vi "ZyklussteuerungGV.vi"(1 "Zeitpunkte/SPs":T2 {"FPGAPID"."proportional gain (Kc)" format="%.11g"; "FPGAPID"."integral gain (Kc*Ts/Ti)" format="%.11g"; "FPGAPID"."derivative gain (Kc*Td/Ts)" format="%.11g"; "FPGAFixp" format="%.14g"}, 2 "DIOsNummern":cluster{"DIOsMod2BNr":i32[]}[](array[cluster]), 3 "Schieberegister":T1, 6 "FPGA VI Reference In":refnum<k20>) -> (0 "Schieberegister":T1)   [LabVIEW 2010]
uses:
  <vilib>/rvi/errors/niLvFpgaWhatHappensToTopLevelVI.ctl
  <vilib>/rvi/interface/common/niFpgaNodeNameForErrorReporting.ctl
  <vilib>/rvi/errors/niLvFpgaAdjustHostInterfaceError.vi
  <vilib>/rvi/interface/nirviReadWriteControl/nirviReadWriteControl.xnode
  C:/Users/HAGAR-IV/Desktop/Zeugs/markus/version feb 2012/FPGA Bitfiles/pertrasgcfpga2_FPGATarget_FPGA-Programm-10_16368CB6.lvbitx
  C:/Users/HAGAR-IV/Desktop/Zeugs/Johnny/pertrasgc fpga/FPGA-Programm-10-14.vi
  GVZwangs.vi
  GVHorstSP.vi
  GVHeizenLH.vi
  GVVentilposition.vi
  GVZeitenZyklen.vi
  NiFpgaLv.dll
  <vilib>/Utility/error.llb/Error Cluster From Error Code.vi
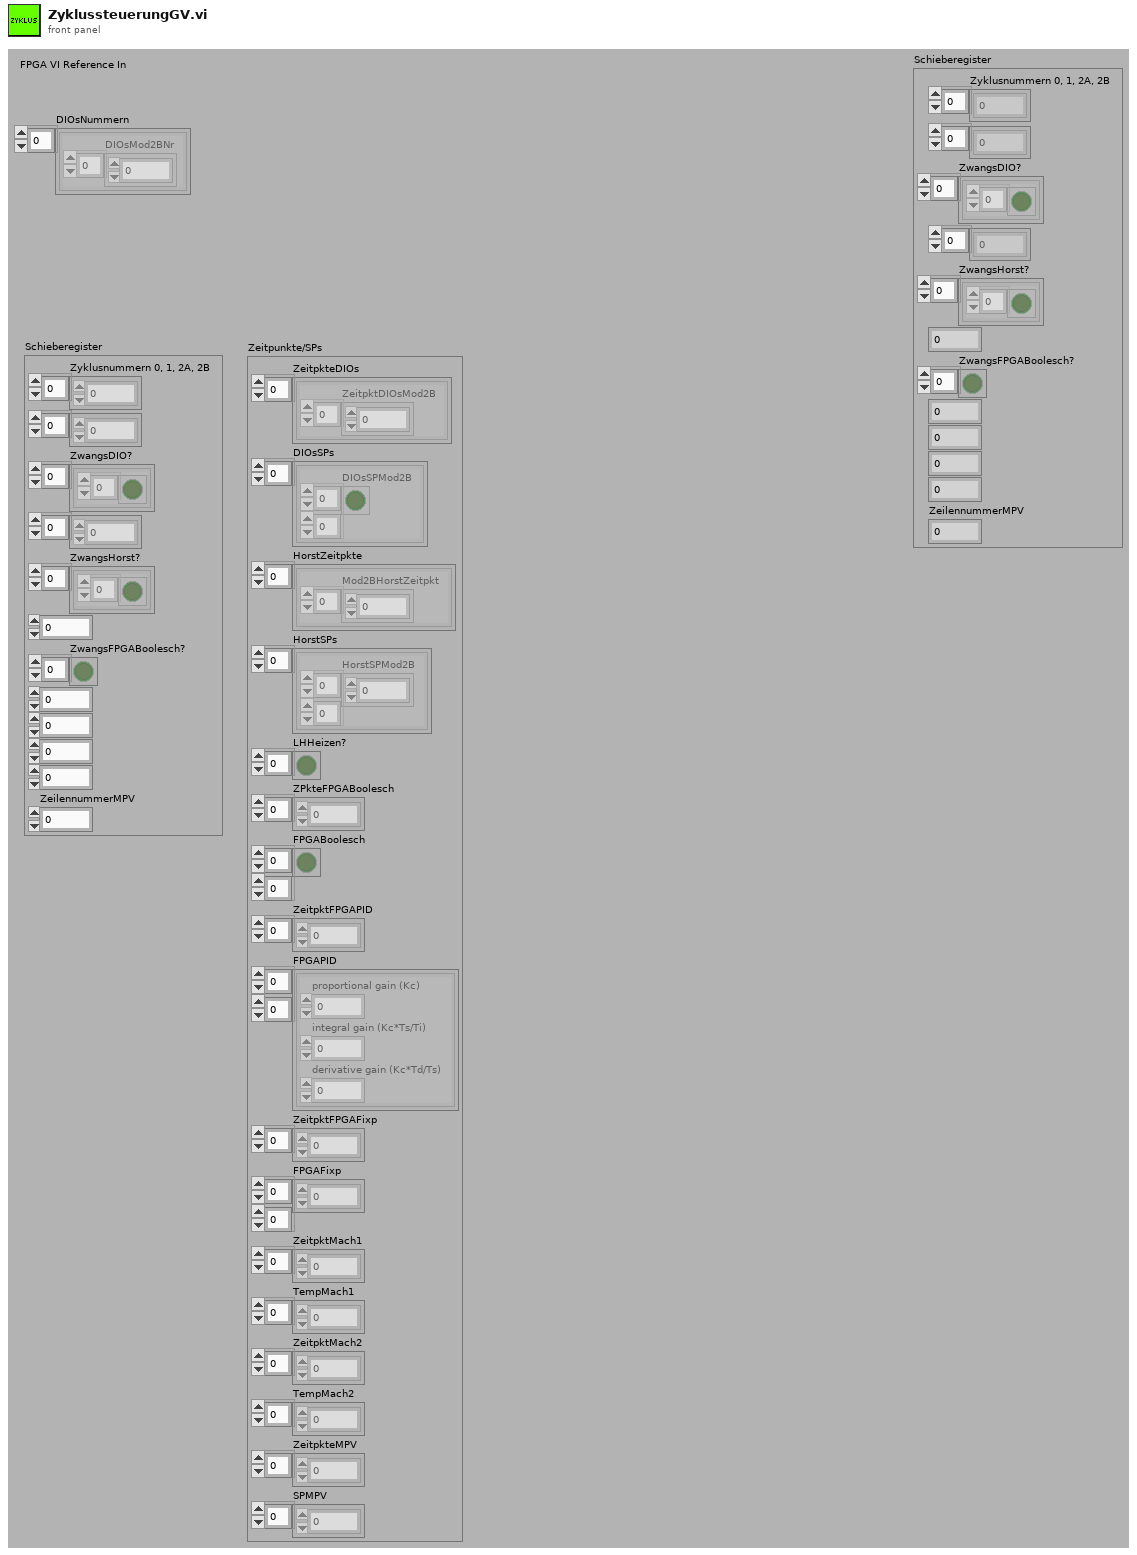
[diagram p1: front panel]
types:
  T1 = cluster{"Zyklusnummern 0, 1, 2A, 2B":i32[], i32[], "ZwangsDIO?":cluster{bool[]}[], i32[], "ZwangsHorst?":cluster{bool[]}[], i32, "ZwangsFPGABoolesch?":bool[], i32, i32, i32, i32, "ZeilennummerMPV":i32}
  T2 = cluster{"ZeitpkteDIOs":cluster{"ZeitpktDIOsMod2B":dbl[]}[], "DIOsSPs":cluster{"DIOsSPMod2B":bool[][]}[], "HorstZeitpkte":cluster{"Mod2BHorstZeitpkt":dbl[]}[], "HorstSPs":cluster{"HorstSPMod2B":dbl[][]}[], "LHHeizen?":bool[], "ZPkteFPGABoolesch":dbl[], "FPGABoolesch":bool[][], "ZeitpktFPGAPID":dbl[], "FPGAPID":cluster{"proportional gain (Kc)":fxp<+/-,16,8>, "integral gain (Kc*Ts/Ti)":fxp<+/-,16,8>, "derivative gain (Kc*Td/Ts)":fxp<+/-,16,8>}[][], "ZeitpktFPGAFixp":dbl[], "FPGAFixp":fxp<+/-,16,4>[][], "ZeitpktMach1":dbl[], "TempMach1":dbl[], "ZeitpktMach2":dbl[], "TempMach2":dbl[], "ZeitpkteMPV":dbl[], "SPMPV":i32[]}
  T3 = cluster{"proportional gain (Kc)":fxp<+/-,16,8>, "integral gain (Kc*Ts/Ti)":fxp<+/-,16,8>, "derivative gain (Kc*Td/Ts)":fxp<+/-,16,8>}[][]
  T4 = typedef "niFpgaNodeNameForErrorReporting.ctl" = enum16{"Open FPGA VI Reference", "Read/Write Control", "Invoke Method: Abort", "Invoke Method: Acknowledge IRQ", "Invoke Method: Download", "Invoke Method: FIFO.Configure", "Invoke Method: FIFO.Read", "Invoke Method: FIFO.Start", "Invoke Method: FIFO.Stop", "Invoke Method: FIFO.Write", "Invoke Method: Reset", "Invoke Method: Run", "Invoke Method: Wait on IRQ", "Close FPGA VI Reference"}
  T5 = typedef "niLvFpgaWhatHappensToTopLevelVI.ctl" = enum16{"top level VI scripted behind XNode", "top level VI inlined behind XNode"}
  T6 = cluster{"FPGAFixp[0]":fxp<+/-,16,4>, "FPGAFixp[1]":fxp<+/-,16,4>, "FPGAFixp[2]":fxp<+/-,16,4>, "FPGAFixp[3]":fxp<+/-,16,4>, "FPGAFixp[4]":fxp<+/-,16,4>, "FPGAFixp[5]":fxp<+/-,16,4>, "FPGAFixp[6]":fxp<+/-,16,4>, "FPGAFixp[7]":fxp<+/-,16,4>}
  T7 = cluster{"proportional gain (Kc)":fxp<+/-,16,8>, "integral gain (Kc*Ts/Ti)":fxp<+/-,16,8>, "derivative gain (Kc*Td/Ts)":fxp<+/-,16,8>}[]
  T8 = cluster{"FPGAPID[0]":cluster{"proportional gain (Kc)":fxp<+/-,16,8>, "integral gain (Kc*Ts/Ti)":fxp<+/-,16,8>, "derivative gain (Kc*Td/Ts)":fxp<+/-,16,8>}, "FPGAPID[1]":cluster{"proportional gain (Kc)":fxp<+/-,16,8>, "integral gain (Kc*Ts/Ti)":fxp<+/-,16,8>, "derivative gain (Kc*Td/Ts)":fxp<+/-,16,8>}, "FPGAPID[2]":cluster{"proportional gain (Kc)":fxp<+/-,16,8>, "integral gain (Kc*Ts/Ti)":fxp<+/-,16,8>, "derivative gain (Kc*Td/Ts)":fxp<+/-,16,8>}, "FPGAPID[3]":cluster{"proportional gain (Kc)":fxp<+/-,16,8>, "integral gain (Kc*Ts/Ti)":fxp<+/-,16,8>, "derivative gain (Kc*Td/Ts)":fxp<+/-,16,8>}}
  T9 = cluster{"proportional gain (Kc)":fxp<+/-,16,8>, "integral gain (Kc*Ts/Ti)":fxp<+/-,16,8>, "derivative gain (Kc*Td/Ts)":fxp<+/-,16,8>}
  T10 = cluster{"[0]":bool, "[1]":bool, "[2]":bool, "[3]":bool, "[4]":bool, "[5]":bool}
  T11 = cluster{"[0]":bool, "[1]":bool, "[2]":bool, "[3]":bool, "[4]":bool, "[5]":bool, "[6]":bool, "[7]":bool, "[8]":bool, "[9]":bool, "[10]":bool, "[11]":bool, "[12]":bool, "[13]":bool, "[14]":bool, "[15]":bool, "[16]":bool, "[17]":bool, "[18]":bool, "[19]":bool, "[20]":bool, "[21]":bool, "[22]":bool, "[23]":bool, "[24]":bool, "[25]":bool, "[26]":bool, "[27]":bool, "[28]":bool, "[29]":bool, "[30]":bool, "[31]":bool}
  T12 = cluster{"ZyklusNummern":i32[], i32[], "ZwangsDIO?":cluster{bool[]}[], i32[], "ZwangsHorst?":cluster{bool[]}[], i32, "ZwangsFPGABoolesch?":bool[], i32, i32, i32, i32, i32}
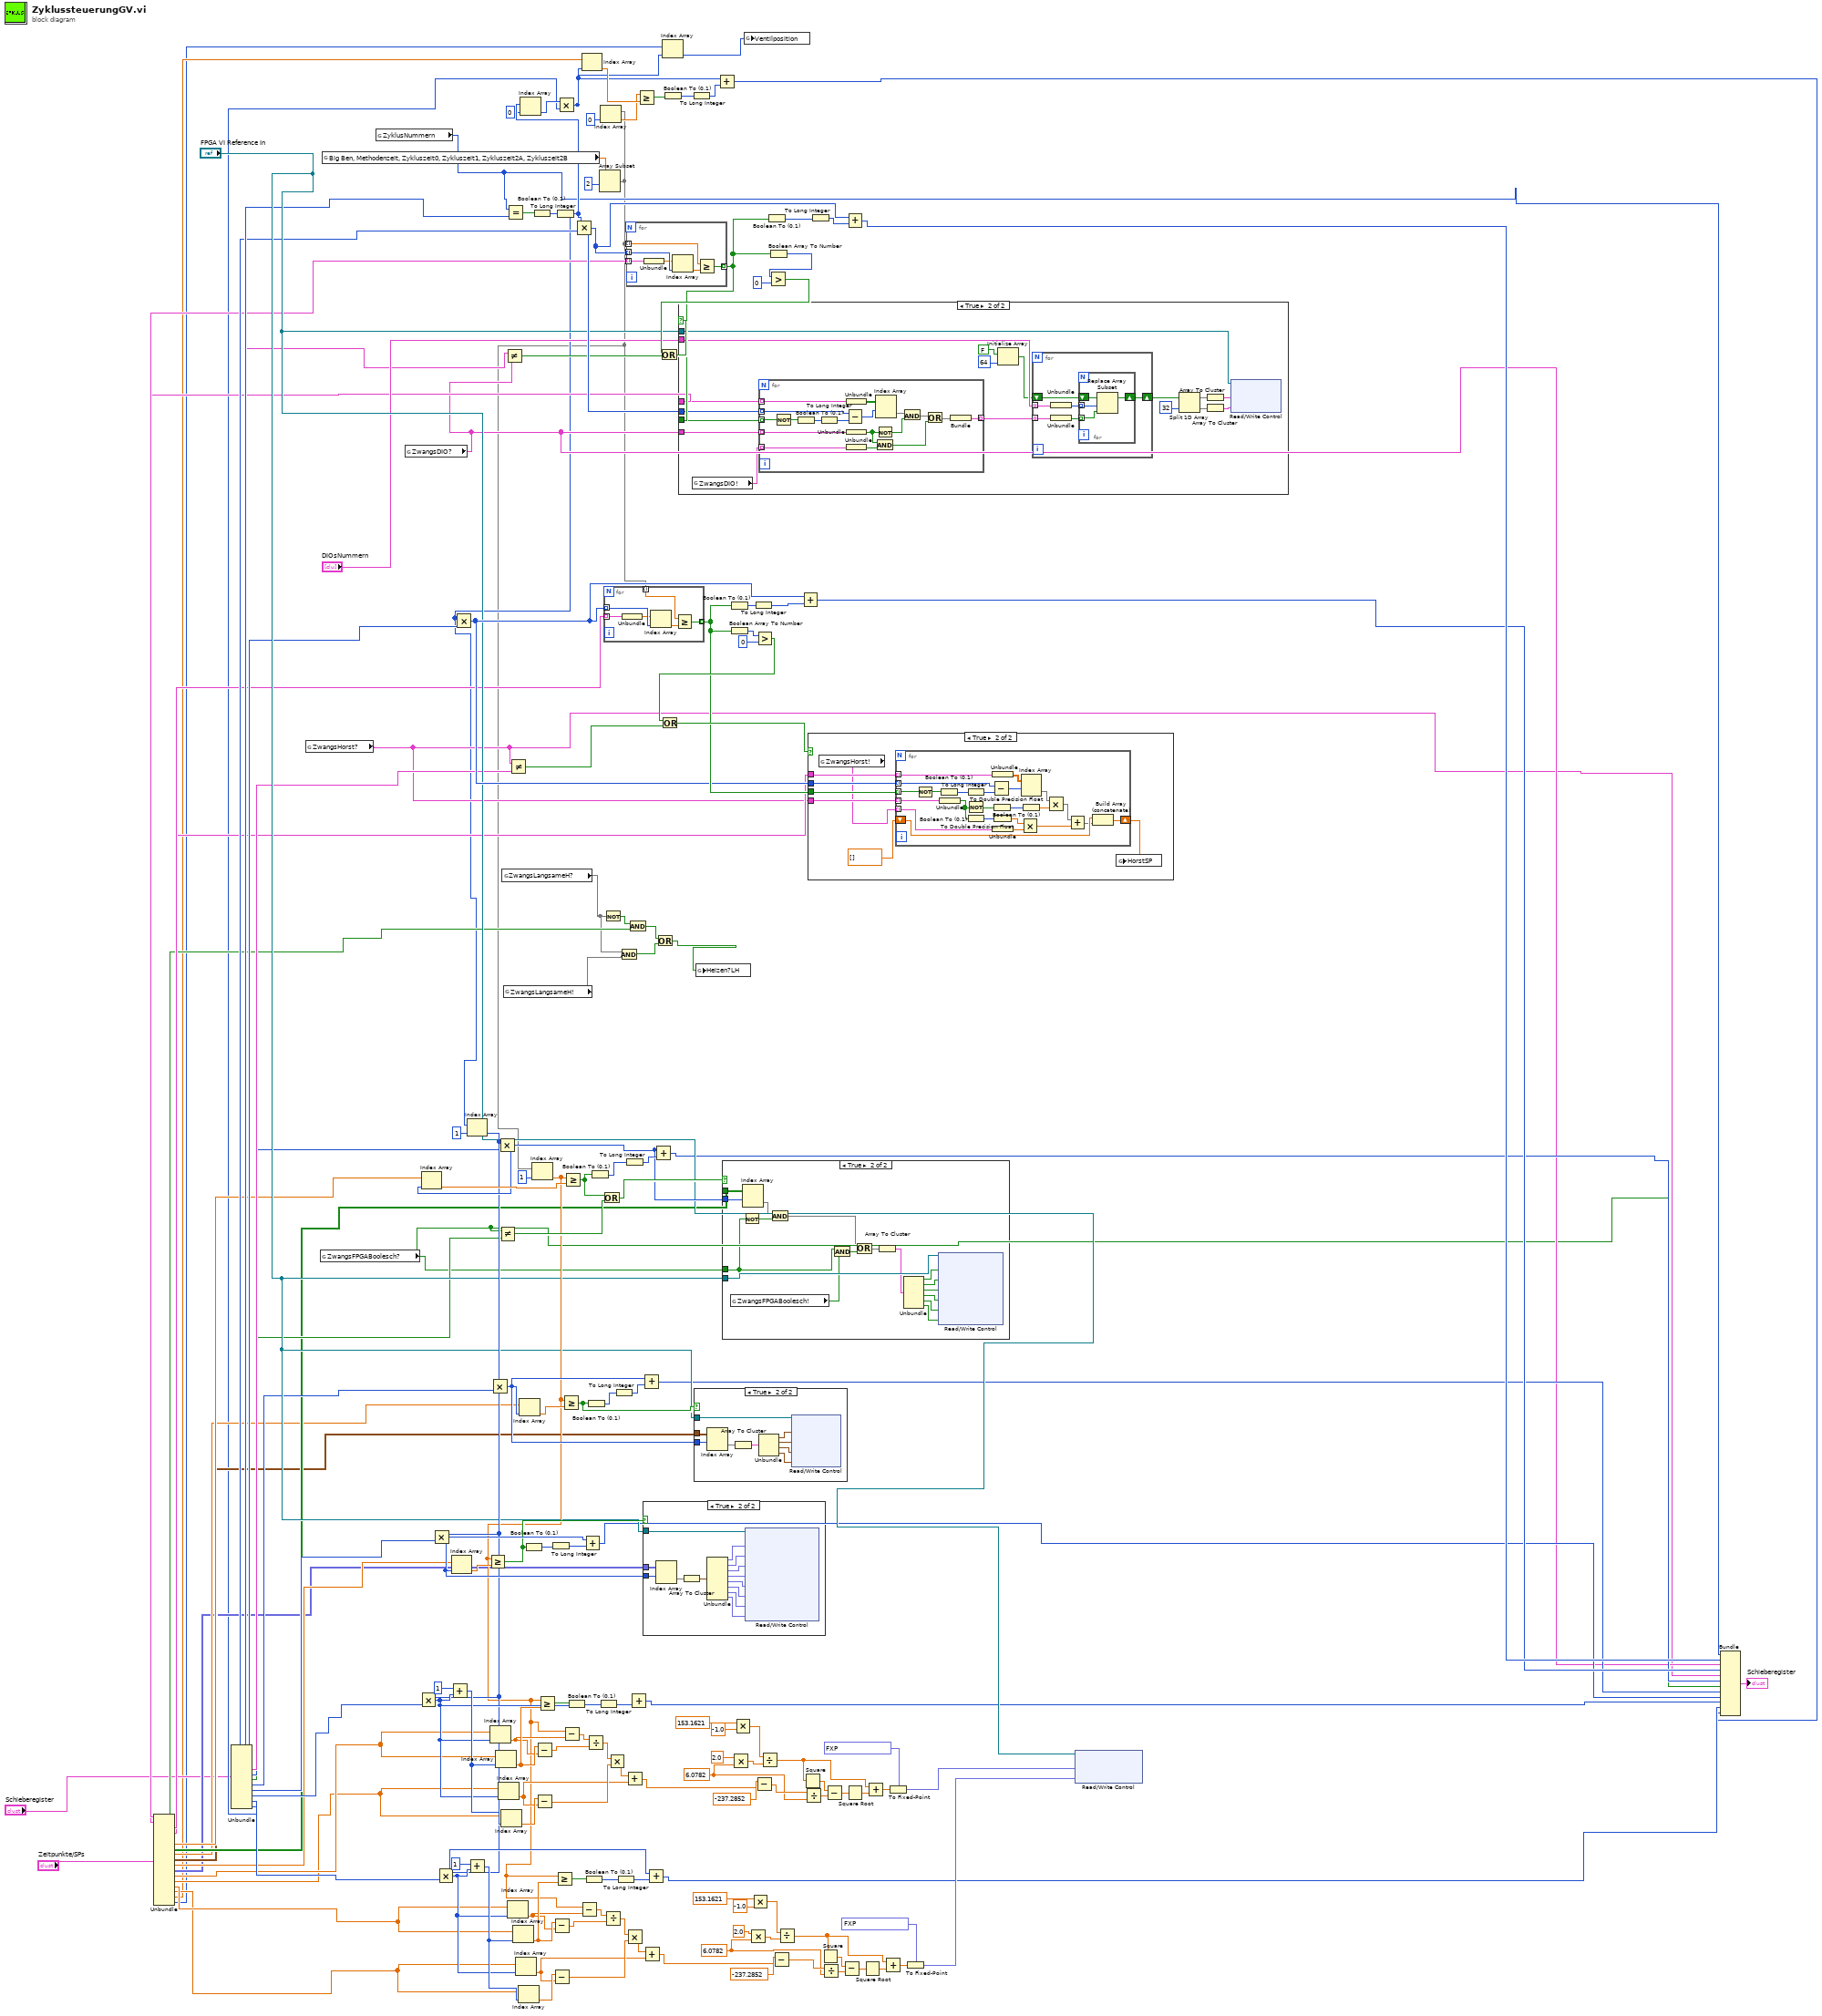
[diagram p0: block diagram]
diagram:
  w82 = 6.0782 ("y")
  w114 = 6.0782 ("y")
  n1 = Unbundle("Zeitpunkte/SPs") -> ("ZeitpkteDIOs"=w43:cluster{"ZeitpktDIOsMod2B":dbl[]}[], "DIOsSPs"=w42:cluster{"DIOsSPMod2B":bool[][]}[], "HorstZeitpkte"=w41:cluster{"Mod2BHorstZeitpkt":dbl[]}[], "HorstSPs"=w40:cluster{"HorstSPMod2B":dbl[][]}[], "LHHeizen?"=w39:bool[], "ZPkteFPGABoolesch"=w38:dbl[], "FPGABoolesch"=w37:bool[][], "ZeitpktFPGAPID"=w36:dbl[], "FPGAPID"=w35:T3, "ZeitpktFPGAFixp"=w34:dbl[], "FPGAFixp"=w33:fxp<+/-,16,4>[][], "ZeitpktMach1"=w32:dbl[], "TempMach1"=w31:dbl[], "ZeitpktMach2"=w30:dbl[], "TempMach2"=w29:dbl[], "ZeitpkteMPV"=w6:dbl[], "SPMPV"=w5:i32[])
  n2 = Unbundle("Schieberegister") -> ("Zyklusnummern 0, 1, 2A, 2B"=w61:i32[], w60:i32[], "ZwangsDIO?"=w59:cluster{bool[]}[], w58:i32[], "ZwangsHorst?"=w57:cluster{bool[]}[], w56:i32, "ZwangsFPGABoolesch?"=w55:bool[], w54:i32, w53:i32, w52:i32, w51:i32, "ZeilennummerMPV"=w9:i32)
  n3 = global read "GVZwangs.vi" "ZwangsHorst?"() -> (w27:cluster{bool[]}[])
  n4 = global read "GVZwangs.vi" "ZwangsFPGABoolesch?"() -> (w23:bool[])
  n5 = global read "GVZeitenZyklen.vi" "Big Ben, Methodenzeit, Zykluszeit0, Zykluszeit1, Zykluszeit2A, Zykluszeit2B"() -> (w2:dbl[])
  n6 = global read "GVZeitenZyklen.vi" "ZyklusNummern"() -> (w4:i32[])
  n7 = global read "GVZwangs.vi" "ZwangsDIO?"() -> (w28:cluster{bool[]}[])
  n8 = Not Equal?(x=w23, y=w55) -> (x != y?=w152:bool)
  n9 = global read "GVZwangs.vi" "ZwangsLangsameH?"() -> (w26)
  n10 = global read "GVZwangs.vi" "ZwangsLangsameH!"() -> (w25)
  n11 = Not Equal?(x=w59, y=w28) -> (x != y?=w66:bool)
  n12 = Equal?(x=w4, y=w61) -> (x = y?=w171:bool[])
  n13 = Not Equal?(x=w27, y=w57) -> (x != y?=w67:bool)
  n14 = Boolean To (0,1)(Boolean=w171) -> (0, 1=w170:i16[])
  n15 = To Long Integer(number=w170) -> (32bit integer=w22:i32[])
  n16 = Multiply(x=w22, y=w58) -> (x*y=w68:i32[])
  n17 = Index Array(array=w22, index=1 ("Index")) -> (element=w79:i32)
  n18 = Multiply(x=w79, y=w52) -> (x*y=w132:i32)
  n19 = Multiply(x=w79, y=w53) -> (x*y=w141:i32)
  n20 = Multiply(x=w79, y=w51) -> (x*y=w102:i32)
  n21 = Add(x=1 ("y"), y=w132) -> (x+y=w138:i32)
  n22 = Index Array(array=w34, index=w141) -> (element=w144:dbl)
  n23 = Add(x=1 ("y"), y=w102) -> (x+y=w108:i32)
  n24 = Multiply(x=w79, y=w54) -> (x*y=w145:i32)
  n25 = Index Array(array=w32, index=w132) -> (element=w131:dbl)
  n26 = Index Array(array=w32, index=w138) -> (element=w136:dbl)
  n27 = Multiply(x=w79, y=w56) -> (x*y=w150:i32)
  n28 = Index Array(array=w38, index=w150) -> (element=w156:dbl)
  n29 = Index Array(array=w31, index=w132) -> (element=w125:dbl)
  n30 = Index Array(array=w31, index=w138) -> (element=w137:dbl)
  n31 = Index Array(array=w30, index=w102) -> (element=w101:dbl)
  n32 = Index Array(array=w30, index=w108) -> (element=w106:dbl)
  n33 = Index Array(array=w29, index=w102) -> (element=w95:dbl)
  n34 = Index Array(array=w29, index=w108) -> (element=w107:dbl)
  n35 = Index Array(array=w36, index=w145) -> (element=w149:dbl)
  n36 = Index Array(array=w22, index=0 ("Index")) -> (element=w20:i32)
  n37 = Subtract(x=w136, y=w131) -> (x-y=w129:dbl)
  n38 = Subtract(x=w137, y=w125) -> (x-y=w127:dbl)
  n39 = Subtract(x=w106, y=w101) -> (x-y=w99:dbl)
  n40 = Subtract(x=w107, y=w95) -> (x-y=w97:dbl)
  n41 = Multiply(x=w20, y=w9) -> (x*y=w13:i32)
  n42 = Multiply(x=w22, y=w60) -> (x*y=w71:i32[])
  n43 = Index Array(array=w6, index=w13) -> (element=w18:dbl)
  n44 = Array Subset(array=w2, index=2 ("Index")) -> (w1:dbl[])  [unwired: 1 in]
  n45 = Index Array(array=w1, index=1 ("Index")) -> (element=w78:dbl)
  n46 = Greater Or Equal?(x=w78, y=w144) -> (x >= y?=w140:bool)
  n47 = Boolean To (0,1)(Boolean=w140) -> (0, 1=w143:i16)
  n48 = Greater Or Equal?(x=w78, y=w136) -> (x >= y?=w135:bool)
  n49 = To Long Integer(number=w143) -> (32bit integer=w142:i32)
  n50 = Greater Or Equal?(x=w78, y=w106) -> (x >= y?=w105:bool)
  n51 = Greater Or Equal?(x=w78, y=w149) -> (x >= y?=w146:bool)
  n52 = Subtract(x=w78, y=w131) -> (x-y=w130:dbl)
  n53 = Greater Or Equal?(x=w78, y=w156) -> (x >= y?=w153:bool)
  n54 = Boolean To (0,1)(Boolean=w135) -> (0, 1=w134:i16)
  n55 = Subtract(x=w78, y=w101) -> (x-y=w100:dbl)
  n56 = Add(x=w141, y=w142) -> (x+y=w46:i32)
  n57 = Boolean To (0,1)(Boolean=w105) -> (0, 1=w104:i16)
  n58 = Boolean To (0,1)(Boolean=w146) -> (0, 1=w148:i16)
  n59 = Divide(x=w130, y=w129) -> (x/y=w128:dbl)
  n60 = Boolean To (0,1)(Boolean=w153) -> (0, 1=w155:i16)
  n61 = To Long Integer(number=w134) -> (32bit integer=w133:i32)
  n62 = Index Array(array=w1, index=0 ("Index")) -> (element=w17:dbl)
  n63 = Or(x=w153, y=w152) -> (x .or. y?=w151:bool)
  n64 = Not(x=w26) -> (.not. x?=w76:bool)
  n65 = Divide(x=w100, y=w99) -> (x/y=w98:dbl)
  n66 = for {
    tunnel: w68 -> [w177] mode=indexing
    tunnel: w1 -> [w176] mode=indexing
    tunnel: w41 -> [w173] mode=indexing
    tunnel: [w174] -> w69 mode=indexing
    n67 = Unbundle(w173) -> ("Mod2BHorstZeitpkt"=w172:dbl[])
    n68 = Index Array(array=w172, index=w177) -> (element=w175:dbl)
    n69 = Greater Or Equal?(x=w176, y=w175) -> (x >= y?=w174:bool)
  }
  n70 = Multiply(x=w128, y=w127) -> (x*y=w126:dbl)
  n71 = To Long Integer(number=w148) -> (32bit integer=w147:i32)
  n72 = To Long Integer(number=w104) -> (32bit integer=w103:i32)
  n73 = And(x=w26, y=w25) -> (x .and. y?=w74:bool)
  n74 = To Long Integer(number=w155) -> (32bit integer=w154:i32)
  n75 = Add(x=w126, y=w125) -> (x+y=w111:dbl)
  n76 = Multiply(x=w98, y=w97) -> (x*y=w96:dbl)
  n77 = for {
    tunnel: w71 -> [w183] mode=indexing
    tunnel: w1 -> [w182] mode=indexing
    tunnel: [w181] -> w65 mode=indexing
    tunnel: w43 -> [w179] mode=indexing
    n78 = Unbundle(w179) -> ("ZeitpktDIOsMod2B"=w178:dbl[])
    n79 = Index Array(array=w178, index=w183) -> (element=w180:dbl)
    n80 = Greater Or Equal?(x=w182, y=w180) -> (x >= y?=w181:bool)
  }
  n81 = And(x=w76, y=w39) -> (x .and. y?=w75:bool[])
  n82 = Add(x=w132, y=w133) -> (x+y=w45:i32)
  n83 = Greater Or Equal?(x=w17, y=w18) -> (x >= y?=w16:bool)
  n84 = Add(x=w145, y=w147) -> (x+y=w47:i32)
  n85 = Add(x=w96, y=w95) -> (x+y=w80:dbl)
  n86 = case shown="True" w140 {
    tunnel: w141 -> [_ w184]
    tunnel: w33 -> [_ w196]
    tunnel: "FPGA VI Reference In" -> [_ w186]
    frame False {
    }
    frame True {
      n87 = Index Array(array=w196, index (row)=w184) -> (element=w185:fxp<+/-,16,4>[])  [unwired: 1 in]
      n88 = Array To Cluster(array=w185) -> (cluster=w195:T6)
      n89 = Unbundle(w195) -> ("FPGAFixp[0]"=w194:fxp<+/-,16,4>, "FPGAFixp[1]"=w193:fxp<+/-,16,4>, "FPGAFixp[2]"=w192:fxp<+/-,16,4>, "FPGAFixp[3]"=w191:fxp<+/-,16,4>, "FPGAFixp[4]"=w190:fxp<+/-,16,4>, "FPGAFixp[5]"=w189:fxp<+/-,16,4>, "FPGAFixp[6]"=w188:fxp<+/-,16,4>, "FPGAFixp[7]"=w187:fxp<+/-,16,4>)
      n90 = xnode "Read/Write Control"("FPGA VI Reference In"=w186, "UTempSPTrap1"=w194, "UTempMaxTrap1"=w193, "UWidrMaxTrap1"=w192, "UTempSPTrap2"=w191, "UTempMaxTrap2"=w190, "UWidrMaxTrap2"=w189, "Umax[V]Mach1"=w188, "Umax[V]Mach2"=w187) -> ()  [unwired: 1 in, 2 out]
    }
  }
  n91 = Add(x=w102, y=w103) -> (x+y=w44:i32)
  n92 = Add(x=w150, y=w154) -> (x+y=w48:i32)
  n93 = Or(x=w75, y=w74) -> (x .or. y?=w24:bool[])
  n94 = Index Array(array=w5, index=w13) -> (element=w12:i32)
  n95 = Boolean To (0,1)(Boolean=w16) -> (0, 1=w15:i16)
  n96 = To Long Integer(number=w15) -> (32bit integer=w14:i32)
  n97 = case shown="True" w146 {
    tunnel: "FPGA VI Reference In" -> [_ w446]
    tunnel: w35 -> [_ w445]
    tunnel: w145 -> [_ w438]
    frame False {
    }
    frame True {
      n98 = Index Array(array=w445, index (row)=w438) -> (element=w444:T7)  [unwired: 1 in]
      n99 = Array To Cluster(array=w444) -> (cluster=w443:T8)
      n100 = Unbundle(w443) -> ("FPGAPID[0]"=w442:T9, "FPGAPID[1]"=w441:T9, "FPGAPID[2]"=w440:T9, "FPGAPID[3]"=w439:T9)
      n101 = xnode "Read/Write Control"("FPGA VI Reference In"=w446, "PIDTrap1"=w442, "PIDTrap2"=w441, "PIDMach1"=w440, "PIDMach2"=w439) -> ()  [unwired: 1 in, 2 out]
    }
  }
  n102 = global write "GVHeizenLH.vi" "Heizen?LH"(w24) -> ()
  n103 = Add(x=w13, y=w14) -> (x+y=w10:i32)
  n104 = case shown="True" w151 {
    tunnel: w150 -> [_ w570]
    tunnel: w23 -> [_ w580]
    tunnel: w37 -> [_ w584]
    tunnel: "FPGA VI Reference In" -> [_ w577]
    frame False {
    }
    frame True {
      n105 = global read "GVZwangs.vi" "ZwangsFPGABoolesch!"() -> (w568:bool[])
      n106 = Not(x=w580) -> (.not. x?=w583:bool[])
      n107 = Index Array(array=w584, index (row)=w570) -> (element=w582:bool[])  [unwired: 1 in]
      n108 = And(x=w582, y=w583) -> (x .and. y?=w581:bool[])
      n109 = And(x=w580, y=w568) -> (x .and. y?=w579:bool[])
      n110 = Or(x=w581, y=w579) -> (x .or. y?=w578:bool[])
      n111 = Array To Cluster(array=w578) -> (cluster=w576:T10)
      n112 = Unbundle(w576) -> ("[0]"=w569:bool, "[1]"=w575:bool, "[2]"=w574:bool, "[3]"=w573:bool, "[4]"=w572:bool, "[5]"=w571:bool)
      n113 = xnode "Read/Write Control"("FPGA VI Reference In"=w577, "ServoTrap1kalt"=w569, "ServoTrap2kalt"=w575, "Heizen?Trap1"=w574, "Heizen?Trap2"=w573, "Heizen?Mach1"=w572, "Heizen?Mach2"=w571) -> ()  [unwired: 1 in, 2 out]
    }
  }
  n114 = Boolean To (0,1)(Boolean=w69) -> (0, 1=w163:i16[])
  n115 = Boolean Array To Number(Boolean array=w69) -> (number=w161:u32)
  n116 = Multiply(x=2.0, y=w114) -> (x*y=w122:dbl)
  n117 = Multiply(x=153.1621 ("y"), y=-1.0) -> (x*y=w123:dbl)
  n118 = global write "GVVentilposition.vi" "Ventilposition"(w12) -> ()
  n119 = Multiply(x=2.0 ("y"), y=w82) -> (x*y=w90:dbl)
  n120 = Multiply(x=153.1621 ("y"), y=-1.0) -> (x*y=w92:dbl)
  n121 = To Long Integer(number=w163) -> (32bit integer=w162:i32[])
  n122 = Subtract(x=-237.2852 ("y"), y=w111) -> (x-y=w119:dbl)
  n123 = Greater?(x=w161, y=u32 0) -> (0:w159:bool)
  n124 = Or(x=w159, y=w67) -> (x .or. y?=w70:bool)
  n125 = Divide(x=w123, y=w122) -> (x/y=w116:dbl)
  n126 = Boolean To (0,1)(Boolean=w65) -> (0, 1=w169:i16[])
  n127 = Boolean Array To Number(Boolean array=w65) -> (number=w167:u32)
  n128 = Greater?(x=w167, y=u32 0) -> (0:w164:bool)
  n129 = Or(x=w164, y=w66) -> (x .or. y?=w165:bool)
  n130 = case shown="True" w165 {
    tunnel: w71 -> [_ w740]
    tunnel: w28 -> [_ w737]
    tunnel: "DIOsNummern" -> [_ w744]
    tunnel: "FPGA VI Reference In" -> [_ w743]
    tunnel: w42 -> [_ w738]
    tunnel: w65 -> [_ w739]
    frame False {
    }
    frame True {
      n131 = global read "GVZwangs.vi" "ZwangsDIO!"() -> (w728:cluster{bool[]}[])
      n132 = for {
        tunnel: w740 -> [w759] mode=indexing
        tunnel: w739 -> [w758] mode=indexing
        tunnel: w738 -> [w757] mode=indexing
        tunnel: w737 -> [w756] mode=indexing
        tunnel: w728 -> [w755] mode=indexing
        tunnel: [w745] -> w736 mode=indexing
        n133 = Not(x=w758) -> (.not. x?=w761:bool)
        n134 = Boolean To (0,1)(Boolean=w761) -> (0, 1=w760:i16)
        n135 = To Long Integer(number=w760) -> (32bit integer=w762:i32)
        n136 = Subtract(x=w759, y=w762) -> (x-y=w753:i32)
        n137 = Unbundle(w757) -> ("DIOsSPMod2B"=w754:bool[][])
        n138 = Unbundle(w756) -> (w750:bool[])
        n139 = Unbundle(w755) -> (w749:bool[])
        n140 = Not(x=w750) -> (.not. x?=w751:bool[])
        n141 = And(x=w750, y=w749) -> (x .and. y?=w747:bool[])
        n142 = Index Array(array=w754, index (row)=w753) -> (element=w752:bool[])  [unwired: 1 in]
        n143 = And(x=w752, y=w751) -> (x .and. y?=w748:bool[])
        n144 = Or(x=w748, y=w747) -> (x .or. y?=w746:bool[])
        n145 = Bundle(w746) -> (w745:cluster{bool[]})  [unwired: 1 in]
      }
      n146 = Initialize Array(FALSE, 64 ("Dimension")) -> (w729:bool[])
      n147 = for {
        tunnel: w736 -> [w837] mode=indexing
        tunnel: w744 -> [w839] mode=indexing
        shift-right: [w840] -> w741
        shift-left: w729 -> [w841]
        n148 = Unbundle(w839) -> ("DIOsMod2BNr"=w838:i32[])
        n149 = Unbundle(w837) -> (w836:bool[])
        n150 = for {
          tunnel: w836 -> [w843] mode=indexing
          tunnel: w838 -> [w844] mode=indexing
          shift-right: [w842] -> w840
          shift-left: w841 -> [w845]
          n151 = Replace Array Subset(array=w845, new element=w843, index=w844) -> (w842:bool[])
        }
      }
      n152 = Split 1D Array(array=w741, index=32 ("Länge")) -> (first subarray=w735:bool[], second subarray=w733:bool[])
      n153 = Array To Cluster(array=w735) -> (cluster=w734:T11)
      n154 = Array To Cluster(array=w733) -> (cluster=w732:T11)
      n155 = xnode "Read/Write Control"("FPGA VI Reference In"=w743, "Mod5/DIO"=w734, "Mod6/DIO"=w732) -> ()  [unwired: 1 in, 2 out]
    }
  }
  n156 = Subtract(x=-237.2852 ("y"), y=w80) -> (x-y=w87:dbl)
  n157 = Divide(x=w92, y=w90) -> (x/y=w84:dbl)
  n158 = Add(x=w68, y=w162) -> (x+y=w49:i32[])
  n159 = Square(x=w116) -> (x^2=w121:dbl)
  n160 = Divide(x=w119, y=w114) -> (x/y=w118:dbl)
  n161 = case shown="True" w70 {
    tunnel: w40 -> [_ w849]
    tunnel: w27 -> [_ w850]
    tunnel: w69 -> [_ w852]
    tunnel: w68 -> [_ w851]
    frame False {
    }
    frame True {
      n162 = global read "GVZwangs.vi" "ZwangsHorst!"() -> (w847:cluster{dbl[]}[])
      n163 = for {
        tunnel: w852 -> [w872] mode=indexing
        tunnel: w851 -> [w869] mode=indexing
        tunnel: w850 -> [w875] mode=indexing
        tunnel: w849 -> [w873] mode=indexing
        tunnel: w847 -> [w874] mode=indexing
        shift-right: [w853] -> w846
        shift-left: dbl[] [] -> [w855]
        n164 = Not(x=w872) -> (.not. x?=w871:bool)
        n165 = Boolean To (0,1)(Boolean=w871) -> (0, 1=w870:i16)
        n166 = Unbundle(w875) -> (w862:bool[])
        n167 = To Long Integer(number=w870) -> (32bit integer=w868:i32)
        n168 = Not(x=w862) -> (.not. x?=w865:bool[])
        n169 = Boolean To (0,1)(Boolean=w862) -> (0, 1=w863:i16[])
        n170 = Subtract(x=w869, y=w868) -> (x-y=w866:i32)
        n171 = Boolean To (0,1)(Boolean=w865) -> (0, 1=w864:i16[])
        n172 = Unbundle(w873) -> ("HorstSPMod2B"=w867:dbl[][])
        n173 = To Double Precision Float(number=w863) -> (double precision float=w859:dbl[])
        n174 = Unbundle(w874) -> (w858:dbl[])
        n175 = Multiply(x=w859, y=w858) -> (x*y=w856:dbl[])
        n176 = Index Array(array=w867, index (row)=w866) -> (element=w861:dbl[])  [unwired: 1 in]
        n177 = To Double Precision Float(number=w864) -> (double precision float=w860:dbl[])
        n178 = Multiply(x=w861, y=w860) -> (x*y=w857:dbl[])
        n179 = Add(x=w857, y=w856) -> (x+y=w854:dbl[])
        n180 = Build Array (concatenate)(w855, w854) -> (w853:dbl[])
      }
      n181 = global write "GVHorstSP.vi" "HorstSP"(w846) -> ()
    }
  }
  n182 = To Long Integer(number=w169) -> (32bit integer=w168:i32[])
  n183 = Square(x=w84) -> (x^2=w89:dbl)
  n184 = Divide(x=w87, y=w82) -> (x/y=w86:dbl)
  n185 = Subtract(x=w121, y=w118) -> (x-y=w117:dbl)
  n186 = Subtract(x=w89, y=w86) -> (x-y=w85:dbl)
  n187 = Add(x=w71, y=w168) -> (x+y=w50:i32[])
  n188 = Square Root(x=w117) -> (sqrt(x)=w115:dbl)
  n189 = Square Root(x=w85) -> (sqrt(x)=w83:dbl)
  n190 = Add(x=w116, y=w115) -> (x+y=w113:dbl)
  n191 = Add(x=w84, y=w83) -> (x+y=w64:dbl)
  n192 = To Fixed-Point(fixed-point type=fxp<+/-,16,4> 0.0 ("USetp [V]Mach1"), number=w113) -> (fixed-point=w110:fxp<+/-,16,4>)
  n193 = To Fixed-Point(fixed-point type=fxp<+/-,16,4> 0.0 ("USetp [V]Mach1"), number=w64) -> (fixed-point=w77:fxp<+/-,16,4>)
  n194 = xnode "Read/Write Control"("FPGA VI Reference In"="FPGA VI Reference In", "USetp[V]Mach1"=w110, "USetp[V]Mach2"=w77) -> ()  [unwired: 1 in, 2 out]
  n195 = Bundle("ZyklusNummern"=w4, w50, "ZwangsDIO?"=w28, w49, "ZwangsHorst?"=w27, w48, "ZwangsFPGABoolesch?"=w23, w47, w46, w45, w44, w10) -> (→"Schieberegister":T12)  [unwired: 1 in]
